vi "PM9840 Control.vi"(8 "error IO":errorcluster, 10 "Address":i8=1, 11 "MyIndex":u8) -> (0 "error OUT":errorcluster caption="error IO", 1 "P":dbl, 2 "I":dbl, 3 "V":dbl)   [LabVIEW 2015]
panel:
  out "VISA":refnum<visa-resource-name> caption="VISA资源名称输出"
  out "StrOut":string
  # "AA01 10CD 4E61 4300 0000 0081 34C3 3C0A D747 4237 39B8 3CFC"
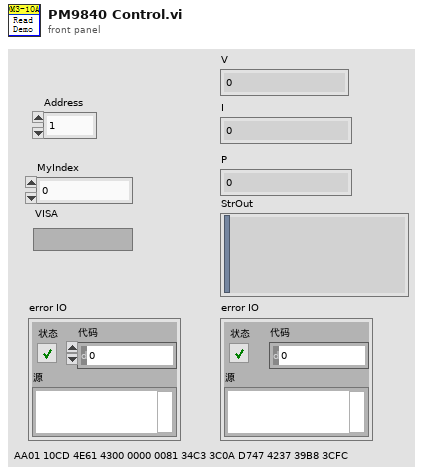
[diagram p1: front panel]
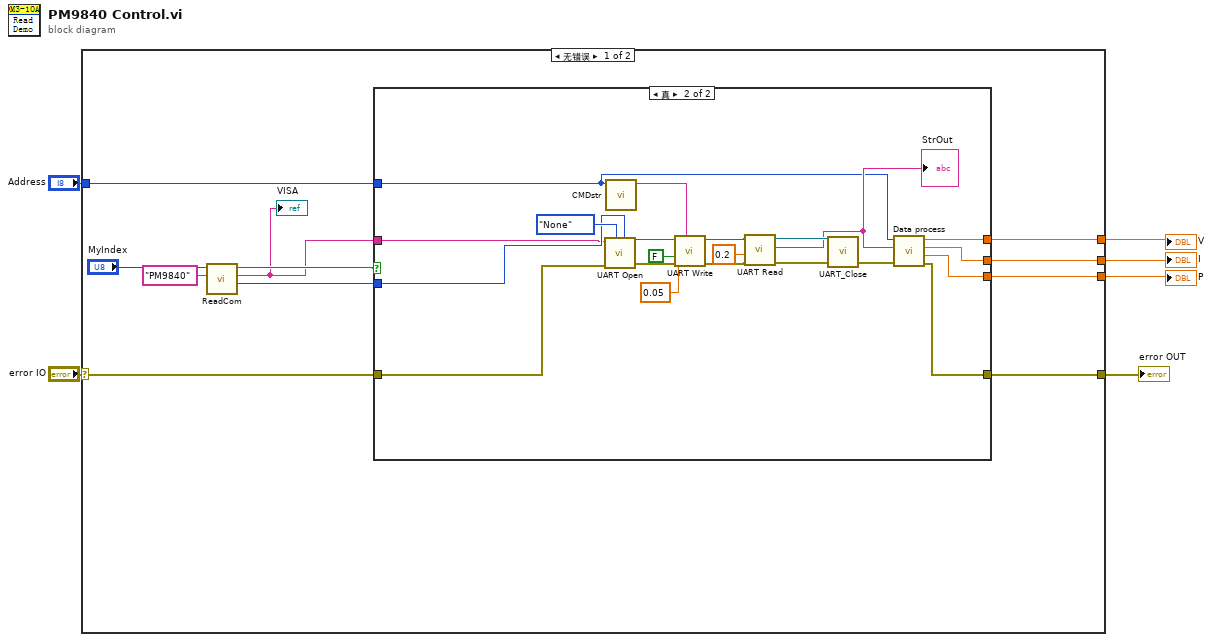
[diagram p0: block diagram]
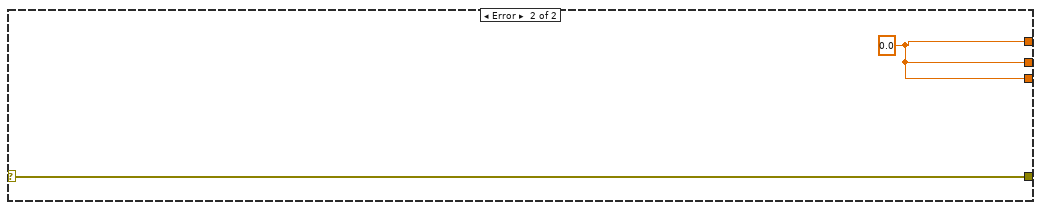
[diagram p3: hidden frame]
diagram:
  n1 = case shown="无错误" "error IO" {
    selector: "error IO" -> [w17 w40]
    tunnel: "Address" -> [w14 _]
    tunnel: [w16 w40] -> w4
    tunnel: [w15 w39] -> w3
    tunnel: [w13 w39] -> w2
    tunnel: [w12 w39] -> w1
    frame No Error {
      n2 = call "ReadCom.vi"("仪器名称"="PM9840", "MyIndex"="MyIndex") -> ("Baudrate"=w8:i32, "COM"=w7:string, "OK?"=w9:bool)  [unwired: 7 in]
      "VISA" <- w7
      n3 = case shown="真" w9 {
        tunnel: w17 -> [_ w38]
        tunnel: [_ w27] -> w16
        tunnel: [_ w24] -> w15
        tunnel: w14 -> [_ w22]
        tunnel: [_ w21] -> w13
        tunnel: [_ w20] -> w12
        tunnel: w8 -> [_ w19]
        tunnel: w7 -> [_ w18]
        frame False {
        }
        frame True {
          n4 = call "UART Open.vi"("baud rate (9600)"=w19, "parity (0:none)"=enum16{"None", "Odd", "Even", "Mark", "Space"}."None", "error in"=w38, "VISA resource name"=w18) -> ("error out"=w37:errorcluster, "VISA resource name out"=w36:refnum<visa-resource-name>)  [unwired: 6 in]
          n5 = call "CMDstr.vi"("Address"=w22) -> ("CMD"=w26:string)  [unwired: 10 in]
          n6 = call "UART Write.vi"("write buffer"=w26, "error in (no error)"=w37, "Add Return"=FALSE, "Write Delay (s)"=0.05, "VISA Resource In"=w36) -> ("error out"=w33:errorcluster, "VISA Resource Out"=w34:refnum<visa-resource-name>)  [unwired: 2 in]
          n7 = call "UART Read.vi"("error in (no error)"=w33, "TimeOut(s)"=0.2, "VISA Resource In"=w34) -> ("error out"=w32:errorcluster, "StrOut"=w25:string, "VISA Resource Out"=w31:refnum<visa-resource-name>)  [unwired: 2 in, 1 out]
          "StrOut" <- w25
          n8 = call "UART_Close.vi"("error in (no error)"=w32, "VISA Resource In"=w31) -> ("error out"=w28:errorcluster)  [unwired: 3 in]
          n9 = call "Data process.vi"("error in"=w28, "Data Read"=w25, "Address"=w22) -> ("error IO"=w27:errorcluster, "P"=w20:dbl, "I"=w21:dbl, "V"=w24:dbl)  [unwired: 5 in]
        }
      }
    }
    frame Error {
      w39 = 0.0 ("Data_Float")
    }
  }
  "error OUT" <- w4
  "V" <- w3
  "I" <- w2
  "P" <- w1
